vi "p4y1.vi"() -> ()   [LabVIEW 2020]
panel:
  in  "file path (use dialog) 2":path
  in  "operation (0:open)":T1(ring)
  in  "access (0:read/write)":enum16{"read/write", "read-only", "write-only"}(ring)
  in  "file path (use dialog)":path
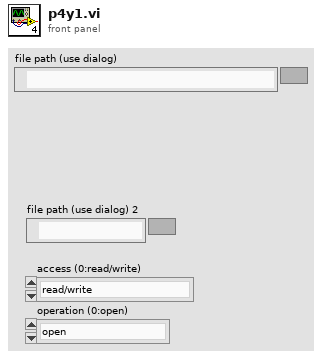
[diagram p1: front panel]
types:
  T1 = enum16{"open", "replace", "create", "open or create", "replace or create", "replace or create with confirmation"}
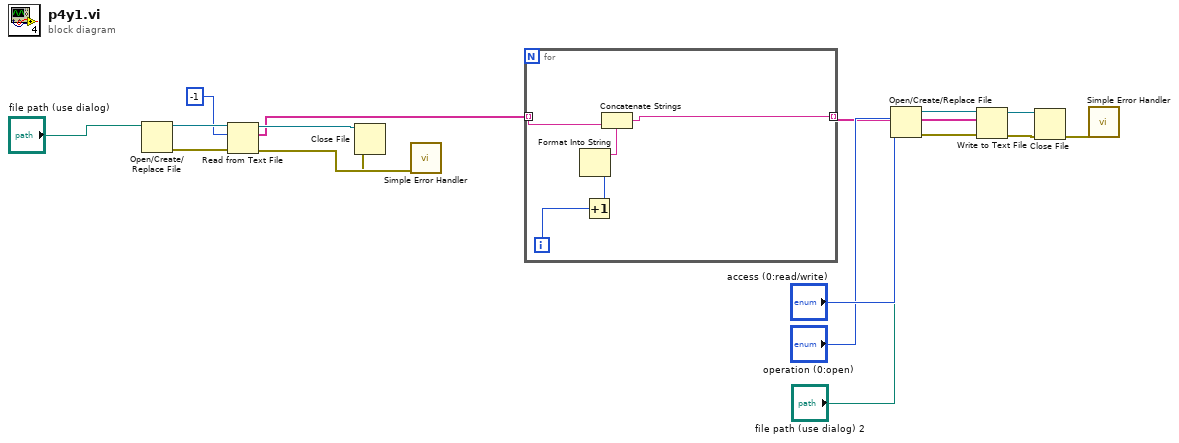
[diagram p0: block diagram]
diagram:
  n1 = Open/Create/Replace File(file path (use dialog)="file path (use dialog)") -> (refnum out=w15:refnum<file>, error out=w17:errorcluster)  [unwired: 5 in, 1 out]
  n2 = Read from Text File(file (use dialog)=w15, count=-1, error in=w17) -> (refnum out=w11:refnum<file>, text=w1:string[], error out=w13:errorcluster)  [unwired: 1 in, 1 out]
  n3 = call <vilib>:"Simple Error Handler.vi"("error in (no error)"=w13) -> ("error out"=w12:errorcluster)  [unwired: 4 in, 4 out]
  n4 = Close File(refnum=w11, error in=w12) -> ()  [unwired: 2 out]
  n5 = for {
    tunnel: w1 -> [w18] mode=indexing
    tunnel: [w20] -> w6 mode=indexing
    i -> [w21]
    n6 = Increment(x=w21) -> (x+1=w22:i32)
    n7 = Format Into String(w22) -> (resulting string=w19:string)  [unwired: 3 in, 1 out]
    n8 = Concatenate Strings(w19, w18) -> (w20:string)
  }
  n9 = Open/Create/Replace File(file path (use dialog)="file path (use dialog) 2", operation (0:open)="operation (0:open)", access (0:read/write)="access (0:read/write)") -> (refnum out=w7:refnum<file>, error out=w5:errorcluster)  [unwired: 3 in, 1 out]
  n10 = Write to Text File(file (use dialog)=w7, text=w6, error in=w5) -> (refnum out=w3:refnum<file>, error out=w4:errorcluster)  [unwired: 1 in, 1 out]
  n11 = Close File(refnum=w3, error in=w4) -> (error out=w2:errorcluster)  [unwired: 1 out]
  n12 = call <vilib>:"Simple Error Handler.vi"("error in (no error)"=w2) -> ()  [unwired: 4 in, 5 out]
